vi "Exp no 2.vi"() -> ()   [LabVIEW 2010]
panel:
  out "Sqrt(X)":dbl
  out "Y-1":dbl
  out "X+1":dbl
  out "X/Y":dbl
  out "X*Y":dbl
  out "X-Y":dbl
  out "X+Y":dbl
  in  "Y":dbl
  in  "X":dbl
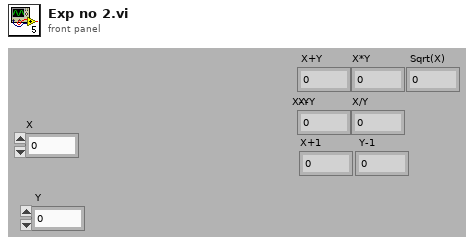
[diagram p1: front panel]
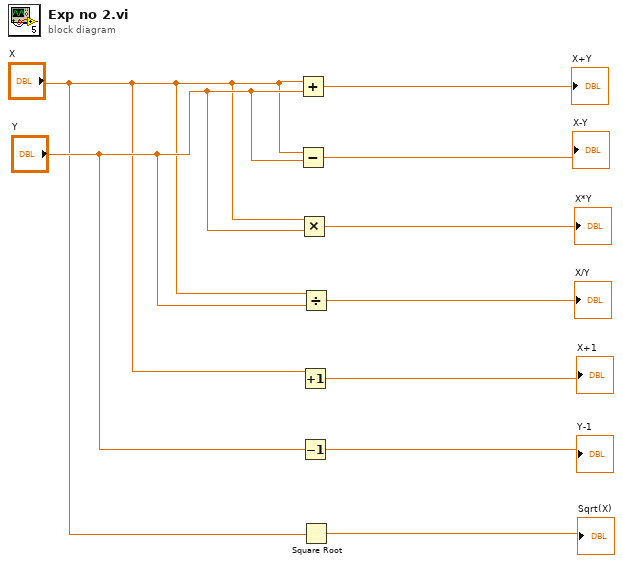
[diagram p0: block diagram]
diagram:
  n1 = Add(x="X", y="Y") -> (x+y=→"X+Y":dbl)
  n2 = Subtract(x="X", y="Y") -> (x-y=→"X-Y":dbl)
  n3 = Multiply(x="X", y="Y") -> (x*y=→"X*Y":dbl)
  n4 = Increment(x="X") -> (x+1=→"X+1":dbl)
  n5 = Decrement(x="Y") -> (x-1=→"Y-1":dbl)
  n6 = Divide(x="X", y="Y") -> (x/y=→"X/Y":dbl)
  n7 = Square Root(x="X") -> (sqrt(x)=→"Sqrt(X)":dbl)
